vi "Simple.vi"() -> ()   [LabVIEW 2016]
panel:
  out "Numeric 5":i32
  out "Boolean out":bool
  in  "Boolean":bool
  out "String out":string
  in  "String":string
  in  "Numeric 12":ext
  in  "Numeric 10":u8
  in  "Numeric 8":i64
  in  "Numeric 6":u64
  in  "Numeric 4":u64
  out "Numeric 3":u64
  in  "stop":bool
  out "Numeric 2":dbl
  in  "Numeric":dbl
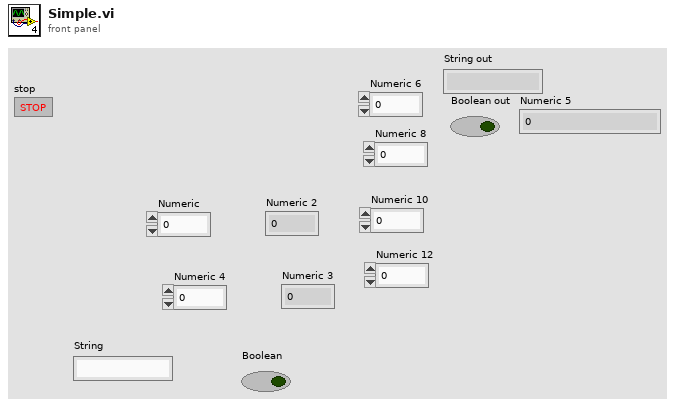
[diagram p1: front panel]
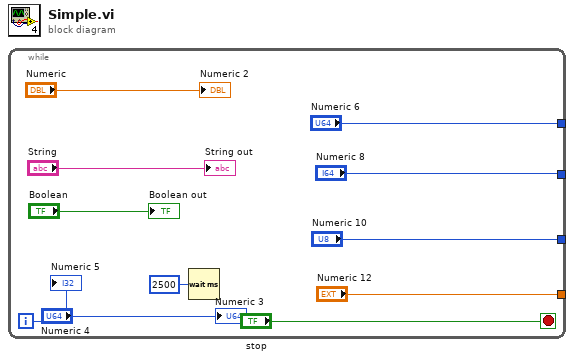
[diagram p0: block diagram]
diagram:
  n1 = while {
    tunnel: ["Numeric 8"] -> _
    tunnel: ["Numeric 10"] -> _
    tunnel: ["Numeric 12"] -> _
    tunnel: ["Numeric 6"] -> _
    i -> [w1]
    stop <- "stop" stop-if-true
    n2 = Wait (ms)(milliseconds to wait=u32 2500) -> ()  [unwired: 1 out]
    "Numeric 2" <- "Numeric"
    "Numeric 3" <- "Numeric 4"
    "String out" <- "String"
    "Boolean out" <- "Boolean"
    "Numeric 5" <- w1
  }
